vi "hdt_int_proto.vi"() -> ()   [LabVIEW 2016]
uses:
  <vilib>/Platform/TimedLoop/XDataNode/timing_clust.ctl
  <vilib>/Platform/TimedLoop/XDataNode/nitl_modes.ctl
  <vilib>/Platform/TimedLoop/XDataNode/wakeup.ctl
  <vilib>/rvi/Emulation/niFpgaGetClockAttributes.vi
  <vilib>/rvi/Emulation/niFpgaSctlEmulationGetInTimedLoop.vi
  <vilib>/rvi/Emulation/niFpgaEmulationReportErrorSimple.vi
  <vilib>/rvi/Emulation/niFpgaEmulationIsFPGAContextNoSignature.vi
  <vilib>/rvi/errors/niFpgaSetErrorForExecOnDevCompSimple.vi
  <vilib>/rvi/eio/common/nirviEmuReportErrorAndStop.vi
  <vilib>/rvi/DataTransferAndStorage/Container/Common/niFpgaContainerGetUniqueNameForEmu.vi
  <vilib>/rvi/FIFO/Fifo_Resource/nirvififoEmulationSetSize.vi
  <vilib>/rvi/FIFO/Fifo_Resource/nirviFifoEmulationQueueMgr.vi
  <instcachedir>/0/nirviFifoEmulationQueueMgr_E5CAEC123FF24DC58D834DCA3CDAA9B5.lvgen/nirviFifoEmulationQueueMgr_E5CAEC123FF24DC58D834DCA3CDAA9B5_014.vi
  <vilib>/Utility/error.llb/Clear Errors.vi
  <vilib>/rvi/FIFO/Fifo_Resource/nirvififoEmulationCreateLock.vi
  <vilib>/rvi/Emulation/niFpgaProcessEmulError.vi
  <vilib>/rvi/FIFO/Fifo_Resource/nirvififoEmulationObtainLock.vi
  <vilib>/rvi/FIFO/Fifo_Resource/nirvififoEmulationReleaseLock.vi
  <vilib>/rvi/occurrence/nirviWaitOnOccurrenceBase.vi
  <vilib>/rvi/errors/nirviReportUnexpectedCaseInternalError.vi
  <vilib>/rvi/errors/nirviReportUnexpectedCaseInternalError (U32).vi
  <vilib>/rvi/interface/RandomDataEmulation/niFpgaRandomDataHandleErrors.vi
  <vilib>/rvi/Emulation/niFpgaCriticalErrorInLSC.vi
  <instcachedir>/0/nirviFifoEmulationQueueMgr_E5CAEC123FF24DC58D834DCA3CDAA9B5.lvgen/nirviFifoEmulationQueueMgr_E5CAEC123FF24DC58D834DCA3CDAA9B5_020.vi
  <vilib>/rvi/FIFO/Fifo_Resource/nirvififoEmulationDetermineInputValidOut.vi
  <vilib>/rvi/Memory/Memory_Emulation/nirvimemoryFastEmulation.vi
  <vilib>/rvi/Memory/Memory_Emulation/nirvimemoryEmulation.vi
  <vilib>/rvi/DataTransferAndStorage/Container/XNode/niFpgaContainer.xnode
  <vilib>/rvi/FIFO/Fifo_Resource/nirvififoEmulationRead.vi
  <vilib>/rvi/interface/RandomDataEmulation/nirviRandomDataFpgaReadWriteTemplate.vi
  <vilib>/Platform/TimedLoop/XDataNode/XDataNode.xnode
  <vilib>/rvi/DataTransferAndStorage/Handshake/Emulation/niFpgaHandshakeEmulation.vi
  <vilib>/rvi/FIFO/Fifo_Resource/nirvififoEmulationWrite.vi
  <vilib>/Platform/TimedLoop/XDataNode/XDNodeRunTimeDep.lvlib
  <instrlib>/_niInstr/Basic Elements/v1/FPGA/niInstr Basic Elements v1 FPGA.lvlib
panel:
  out "hdt.int.s.debug":T1
  out "hdt.int.s.currentStagingEl":cluster{"Element":i16, "Output Valid":bool}
  in  "hdt.int.p.readParams":T2={"hdt.int.s.transferSource"=0, "hdt.int.p.useInternalMemStartPos"=FALSE, "hdt.int.p.memStartPos"=0, "hdt.int.p.readLength"=0, "hdt.int.p.memReadDec"=10, "hdt.int.p.startTransfer"=TRUE} {"hdt.int.s.transferSource" items=["memoryChan1", "memoryChan2", "processVarFixedNoPts", "processVarStream"]}
  out "hdt.int.s.storedMemPos":u16
  in  "hdt.int.p.memWriteSource":u8(ring) items=["ORT", "SICM"]
  out "hdt.int.s.dataLost":bool
  in  "hdt.int.s.clearDataLost":bool
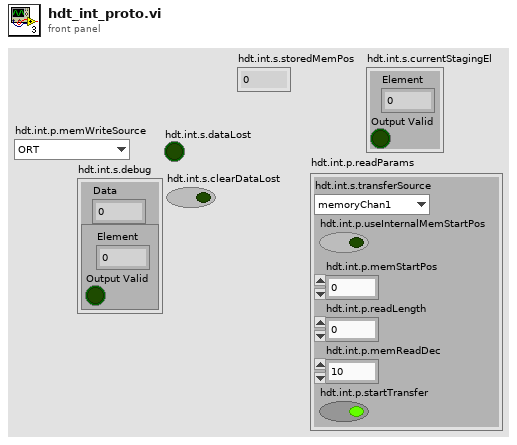
[diagram p1: front panel]
types:
  T1 = cluster{"Data":u16, cluster{"Element":i16, "Output Valid":bool}}
  T2 = cluster{"hdt.int.s.transferSource":u8, "hdt.int.p.useInternalMemStartPos":bool, "hdt.int.p.memStartPos":u16, "hdt.int.p.readLength":u16, "hdt.int.p.memReadDec":u16, "hdt.int.p.startTransfer":bool}
  T3 = typedef "XDNodeRunTimeDep.lvlib/timing_clust.ctl" = cluster{"Expected End [f-1]":u64, "Actual End [f-1]":u64, "Finished Late? [f-1]":bool, "Expected End [i-1]":u64, "Actual End [i-1]":u64, "Finished Late? [i-1]":bool, "Expected Start [i]":u64, "Actual Start [i]":u64, "Expected Start [f]":u64, "Actual Start [f]":u64, "Source Name":string, "Structure Name":string, "Period":i64, "Deadline":i64, "Offset":i64, "Start":i64, "Priority":i32, "Timeout":i32, "Mode":T4, "Wakeup Reason":T5, "Error":errorcluster, "Source Type":string, "Secondary Source Type":string, "Global End Time":u64, "Global Start Time":u64, "Frame Duration":u64, "Iteration Duration":u64, "Assigned CPU":i32, "I/O Scan Engine Mode":u32}
  T4 = typedef "XDNodeRunTimeDep.lvlib/nitl_modes.ctl" = enum32{"No Change", "Process missed periods, maintain original phase", "Discard missed periods, maintain original phase", "Process missed periods, ignore original phase", "Discard missed periods, ignore original phase"}
  T5 = typedef "XDNodeRunTimeDep.lvlib/wakeup.ctl" = enum32{"Normal", "Aborted", "Asynchronous wakeup", "Timing source error", "Timed loop error", "Timeout"}
  T6 = cluster{"address":u16, "interactionPair":cluster{"interaction":i16, "background":i16}}
  T7 = cluster{"Element":cluster{"address":u16, "interactionPair":cluster{"interaction":i16, "background":i16}}, "Output Valid":bool}
  T8 = cluster{"Element":cluster{"address":u16, "interactionPair":cluster{"interaction":i16, "background":i16}}, "Output Valid":bool}[]
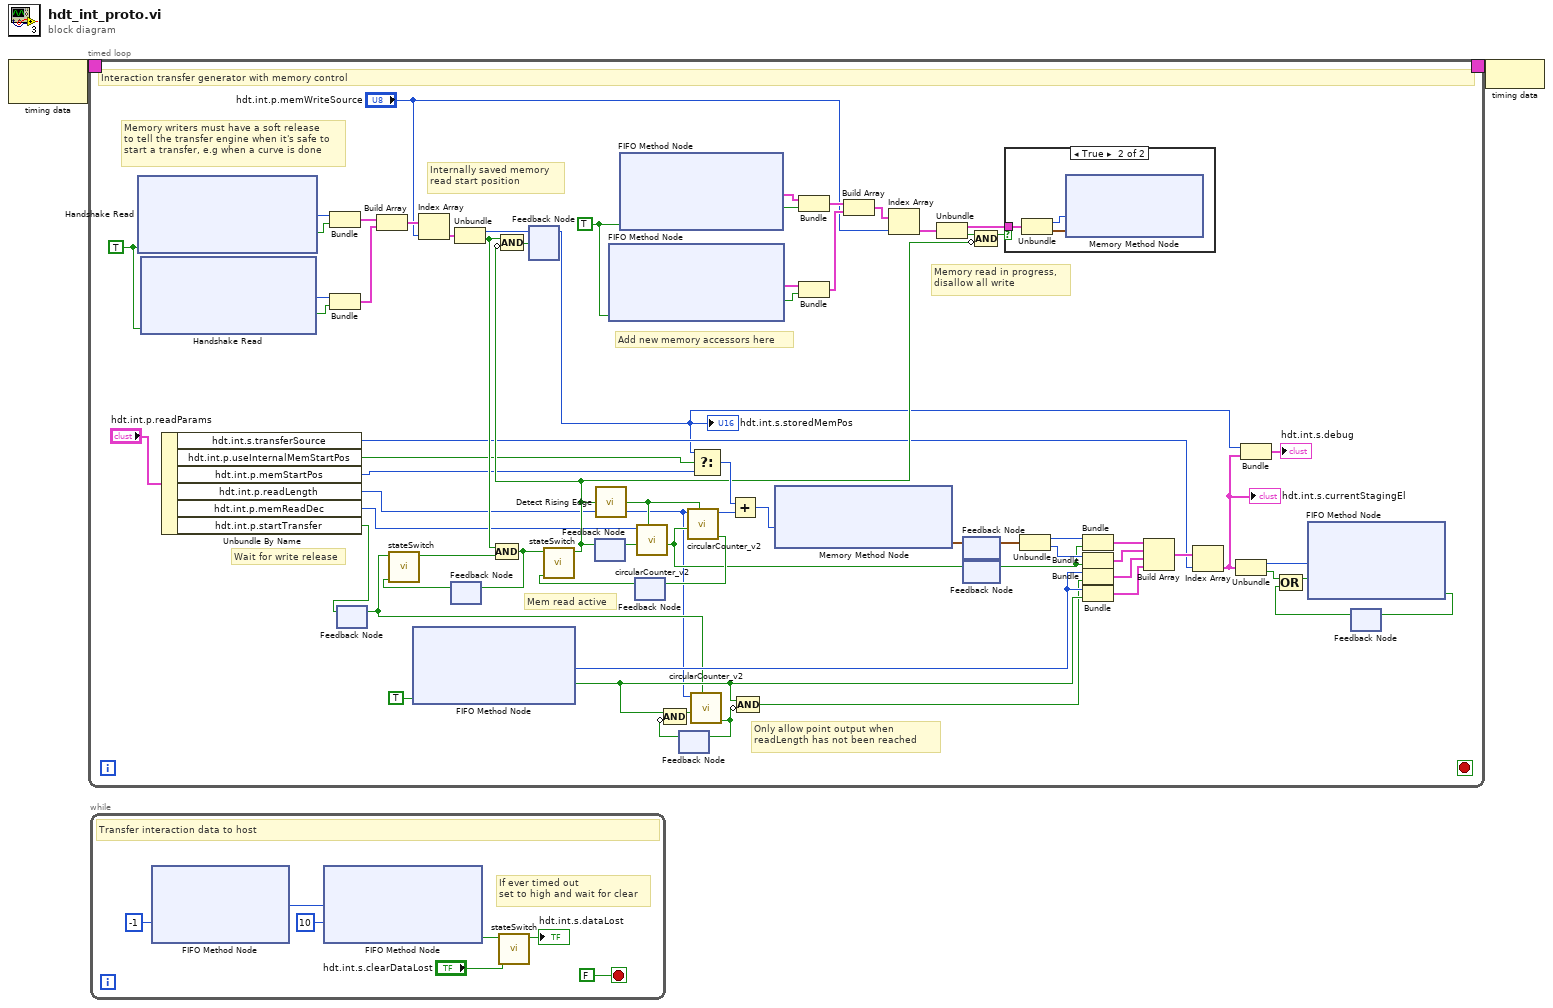
[diagram p0: block diagram]
diagram:
  n1 = node-c288() -> (w2:T3)  [unwired: 1 in]
  n2 = timed-loop {
    timing: w2 -> [_]
    timing-out: [_] -> w1
    stop <- _ stop-if-true
    w19 = TRUE ("Ready for Output")
    w20 = TRUE ("Ready for Output")
    # "Mem read active"
    # "Internally saved memory \nread start position"
    # "Memory writers must have a soft release\nto tell the transfer engine when it's safe to\nstart a transfer, e.g when a curve is done"
    # "Wait for write release"
    # "Only allow point output when readLength has not been reached"
    # "Memory read in progress,\ndisallow all write"
    # "Add new memory accessors here"
    # "Interaction transfer generator with memory control"
    n3 = xnode "Handshake Read"("Ready for Output"=w19) -> ("Data"=w31:u16, "Output Valid"=w30:bool)  [unwired: 1 in, 1 out]
    n4 = xnode "Handshake Read"("Ready for Output"=w19) -> ("Data"=w33:u16, "Output Valid"=w32:bool)  [unwired: 1 in, 1 out]
    n5 = Unbundle By Name("hdt.int.p.readParams") -> ("hdt.int.s.transferSource"=w11:u8, "hdt.int.p.useInternalMemStartPos"=w9:bool, "hdt.int.p.memStartPos"=w10:u16, "hdt.int.p.readLength"=w8:u16, "hdt.int.p.memReadDec"=w7:u16, "hdt.int.p.startTransfer"=w6:bool)
    n6 = Bundle("Data"=w31, "Output Valid"=w30) -> (w29:cluster{"Data":u16, "Output Valid":bool})  [unwired: 1 in]
    n7 = Bundle("Data"=w33, "Output Valid"=w32) -> (w28:cluster{"Data":u16, "Output Valid":bool})  [unwired: 1 in]
    n8 = feedback-in #1(w6) -> ()
    n9 = feedback #1() -> (w13:bool)  [unwired: 1 in]
    n10 = Build Array(w29, w28) -> (w27:cluster{"Data":u16, "Output Valid":bool}[])
    n11 = xnode ("FIFO Method Node")("Ready for Output"=TRUE) -> ("Element"=w41:i16, "Output Valid"=w36:bool)  [unwired: 1 in, 1 out]
    n12 = Index Array(array=w27, index="hdt.int.p.memWriteSource") -> (element=w25:cluster{"Data":u16, "Output Valid":bool})
    n13 = feedback #2() -> (w21:bool)  [unwired: 1 in]
    n14 = call "stateSwitch.vi"("disable"=w21, "enable"=w13) -> ("state"=w23:bool)  [unwired: 9 in]
    n15 = Unbundle(w25) -> ("Data"=w24:u16, "Output Valid"=w16:bool)
    n16 = Compound Arithmetic op=AND(w16, w23) -> (w22:bool)
    n17 = feedback-in #2(w22) -> ()
    n18 = feedback #3() -> (w4:u16)  [unwired: 1 in]
    "hdt.int.s.storedMemPos" <- w4
    n19 = feedback #4() -> (w17:bool)  [unwired: 1 in]
    n20 = xnode ("FIFO Method Node")("Ready for Output"=w20) -> ("Element"=w64:T6, "Output Valid"=w63:bool)  [unwired: 1 in, 1 out]
    n21 = xnode ("FIFO Method Node")("Ready for Output"=w20) -> ("Element"=w71:T6, "Output Valid"=w70:bool)  [unwired: 1 in, 1 out]
    n22 = feedback #5() -> (w50:bool)  [unwired: 1 in]
    n23 = call "stateSwitch.vi"("disable"=w50, "enable"=w22) -> ("state"=w15:bool)  [unwired: 9 in]
    n24 = Compound Arithmetic op=AND(w16, invert w15) -> (w14:bool)
    n25 = feedback-in #3(w24, w14) -> ()
    n26 = feedback-in #4(w15) -> ()
    n27 = call <instrlib>:"Detect Rising Edge.vi"("signal"=w15) -> ("edge detected"=w18:bool)  [unwired: 14 in]
    n28 = call "circularCounter_v2.vi"("reset"=w18, "doStep"=w17, "maxCount"=w7) -> ("maxPulse"=w48:bool)  [unwired: 5 in, 3 out]
    n29 = feedback #6() -> (w38:bool)  [unwired: 1 in]
    n30 = Compound Arithmetic op=AND(w36, invert w38) -> (w39:bool)
    n31 = call "circularCounter_v2.vi"("reset"=w18, "doStep"=w48, "maxCount"=w8) -> ("maxReached"=w51:bool, "index"=w53:u16)  [unwired: 5 in, 2 out]
    n32 = feedback-in #5(w51) -> ()
    n33 = call "circularCounter_v2.vi"("reset"=w13, "doStep"=w39, "maxCount"=w8) -> ("maxReached"=w37:bool)  [unwired: 5 in, 3 out]
    n34 = feedback-in #6(w37) -> ()
    n35 = Select(t=w4, s=w9, f=w10) -> (s? t:f=w34:u16)
    n36 = Add(x=w34, y=w53) -> (x+y=w52:u16)
    n37 = Compound Arithmetic op=AND(w36, invert w37) -> (w35:bool)
    n38 = xnode ("Memory Method Node")("Address"=w52) -> ("Data"=w60:cluster{"interaction":i16, "background":i16})  [unwired: 1 in, 1 out]
    n39 = Bundle("Element"=w71, "Output Valid"=w70) -> (w69:T7)  [unwired: 1 in]
    n40 = Bundle("Element"=w64, "Output Valid"=w63) -> (w62:T7)  [unwired: 1 in]
    n41 = Build Array(w69, w62) -> (w72:T8)
    n42 = Index Array(array=w72, index="hdt.int.p.memWriteSource") -> (element=w68:T7)
    n43 = Unbundle(w68) -> ("Element"=w66:T6, "Output Valid"=w67:bool)
    n44 = feedback-in #7(w60) -> ()
    n45 = feedback #7() -> (w49:cluster{"interaction":i16, "background":i16})  [unwired: 1 in]
    n46 = feedback #8() -> (w47:bool)  [unwired: 1 in]
    n47 = feedback-in #8(w48) -> ()
    n48 = Compound Arithmetic op=AND(w67, invert w15) -> (w65:bool)
    n49 = case shown="True" w65 {
      tunnel: w66 -> [_ w75]
      frame False {
      }
      frame True {
        n50 = Unbundle(w75) -> ("address"=w74:u16, "interactionPair"=w73:cluster{"interaction":i16, "background":i16})
        n51 = xnode ("Memory Method Node")("Address"=w74, "Data"=w73) -> ()  [unwired: 1 in, 1 out]
      }
    }
    n52 = Unbundle(w49) -> ("interaction"=w59:i16, "background"=w58:i16)
    n53 = Bundle("interaction"=w59, "maxPulse"=w47) -> (w57:cluster{"interaction":i16, "maxPulse":bool})  [unwired: 1 in]
    n54 = Bundle("background"=w58, "maxPulse"=w47) -> (w56:cluster{"background":i16, "maxPulse":bool})  [unwired: 1 in]
    n55 = Bundle("Element"=w41, w35) -> (w43:cluster{"Element":i16, bool})  [unwired: 1 in]
    n56 = Bundle("Element"=w41, "Output Valid"=w36) -> (w40:cluster{"Element":i16, "Output Valid":bool})  [unwired: 1 in]
    n57 = Build Array(w57, w56, w43, w40) -> (w61:cluster{"Element":i16, "Output Valid":bool}[])
    n58 = Index Array(array=w61, index=w11) -> (element=w5:cluster{"Element":i16, "Output Valid":bool})
    "hdt.int.s.currentStagingEl" <- w5
    n59 = Unbundle(w5) -> ("Element"=w55:i16, "Output Valid"=w54:bool)
    n60 = Bundle("Data"=w4, w5) -> (→"hdt.int.s.debug":T1)  [unwired: 1 in]
    n61 = feedback #9() -> (w44:bool)  [unwired: 1 in]
    n62 = Compound Arithmetic op=OR(w54, w44) -> (w46:bool)
    n63 = xnode ("FIFO Method Node")("Element"=w55, "Input Valid"=w46) -> ("Ready for Input"=w45:bool)  [unwired: 1 in, 1 out]
    n64 = feedback-in #9(w45) -> ()
  }
  n65 = while {
    stop <- FALSE stop-if-true
    # "If ever timed out\nset to high and wait for clear"
    # "Transfer interaction data to host"
    n66 = xnode ("FIFO Method Node")("Timeout"=-1) -> ("Element"=w83:i16)  [unwired: 1 in, 2 out]
    n67 = xnode ("FIFO Method Node")("Element"=w83, "Timeout"=10) -> ("Timed Out?"=w81:bool)  [unwired: 1 in, 1 out]
    n68 = call "stateSwitch.vi"("disable"="hdt.int.s.clearDataLost", "enable"=w81) -> ("state"=→"hdt.int.s.dataLost":bool)  [unwired: 9 in]
  }
  n69 = node-c288(w1) -> ()
